vi "ActiveObjects_QueueQueue_SendMsgToProcess_6x8x6.vi"(0 "reference in":refnum<class>, 2 "MessageToProcess":string, 5 "Error In":errorcluster) -> (14 "reference out":refnum<class>, 19 "Error Out":errorcluster)   [LabVIEW 2020]
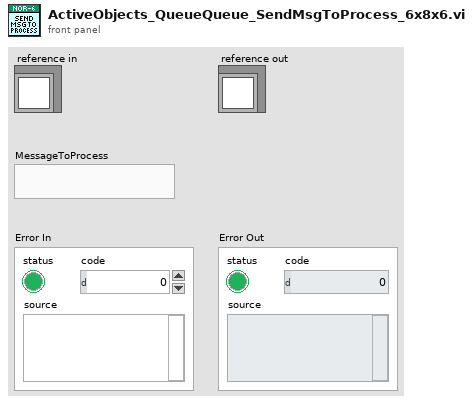
[diagram p1: front panel]
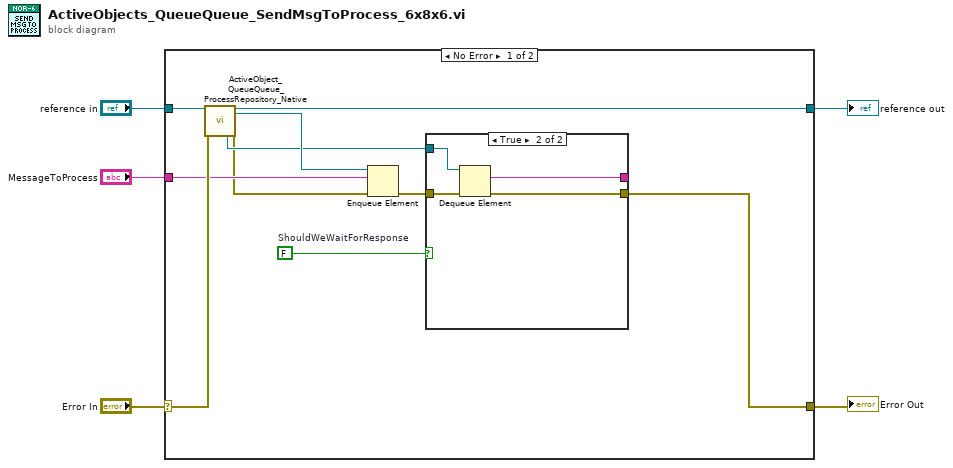
[diagram p0: block diagram]
diagram:
  n1 = case shown="No Error" "Error In" {
    selector: "Error In" -> [w15 w22]
    tunnel: [w6 w22] -> w4
    tunnel: [w13 w21] -> w2
    tunnel: "reference in" -> [w14 w21]
    tunnel: "MessageToProcess" -> [w11 _]
    frame No Error {
      w10 = FALSE  # ShouldWeWaitForResponse
      n2 = call "ActiveObject_QueueQueue_ProcessRepository_Native.vi"("reference in"=w14, "Error In"=w15) -> ("FromProcessQueue"=w8:refnum<queue>, "reference out"=w13:refnum<class>, "ToProcessQueue"=w12:refnum<queue>, "Error Out"=w7:errorcluster)  [unwired: 11 in, 3 out]
      n3 = Enqueue Element(queue=w12, element=w11, error in (no error)=w7) -> (error out=w9:errorcluster)  [unwired: 1 in, 2 out]
      n4 = case shown="True" w10 {
        tunnel: w9 -> [w16 w20]
        tunnel: w8 -> [_ w19]
        tunnel: [_ w18] -> _
        tunnel: [w16 w17] -> w6
        frame False {
        }
        frame True {
          n5 = Dequeue Element(queue=w19, error in (no error)=w20) -> (element=w18:string, error out=w17:errorcluster)  [unwired: 1 in, 2 out]
        }
      }
    }
    frame Error {
    }
  }
  "Error Out" <- w4
  "reference out" <- w2
